vi "Exp1.vi"() -> ()   [LabVIEW 2018]
uses:
  <vilib>/Platform/TimedLoop/XDataNode/timing_clust.ctl
  <vilib>/Platform/TimedLoop/XDataNode/nitl_modes.ctl
  <vilib>/Platform/TimedLoop/XDataNode/wakeup.ctl
  <vilib>/MakerHub/LINX/Public/Peripherals/Analog/Analog Read 1 Chan.vi
  <vilib>/MakerHub/LINX/Public/Peripherals/PWM/PWM Set Duty Cycle 1 Chan.vi
  <vilib>/MakerHub/LINX/Public/Peripherals/Analog/Analog Read N Chans.vi
  <vilib>/MakerHub/LINX/Private/Local IO/LinxAnalogRead.vi
  <vilib>/MakerHub/LINX/Public/Utilities/Check Channel.vi
  <vilib>/MakerHub/LINX/Public/Utilities/Open Serial.vi
  <vilib>/MakerHub/LINX/Private/Utilties/Generate Error.vi
  <vilib>/MakerHub/LINX/Public/Peripherals/PWM/PWM Set Duty Cycle N Chans.vi
  <vilib>/platform/TimedLoop/XDataNode/XDataNode.xnode
  <vilib>/MakerHub/LINX/LMH-LINX.lvlib
  <vilib>/Platform/TimedLoop/XDataNode/XDNodeRunTimeDep.lvlib
panel:
  out "Finished Late? [i-1]":bool
  in  "Duty Cycle (0-100)":dbl min=0.0 max=1.0 step=0.1
  out "Temperature":dbl(graph)=297.8515625
  in  "Stop Button":bool
  in  "Serial Port":refnum<visa-resource-name>="COM4"
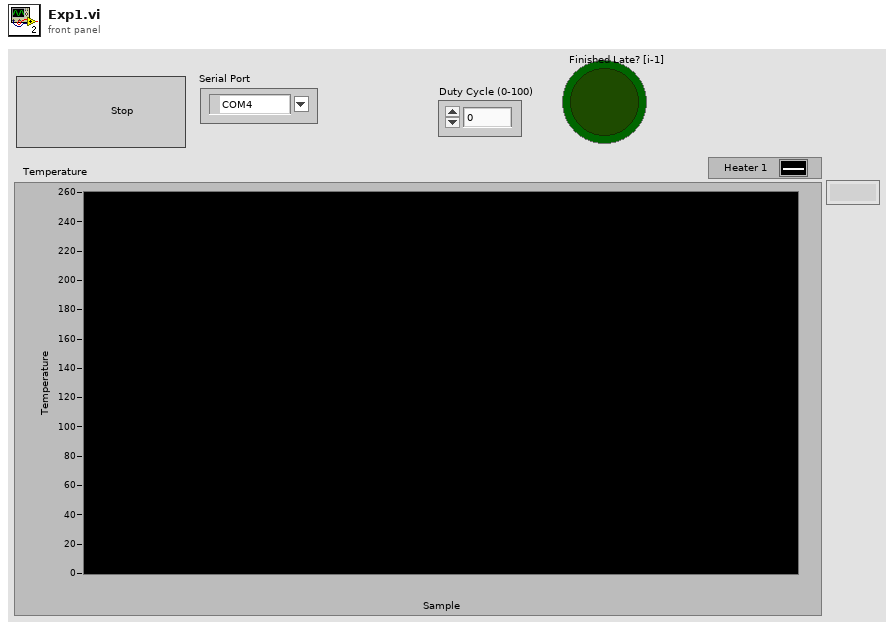
[diagram p1: front panel]
types:
  T1 = enum16{"open", "replace", "create", "open or create", "replace or create", "replace or create with confirmation"}
  T2 = typedef "XDNodeRunTimeDep.lvlib/timing_clust.ctl" = cluster{"Expected End [f-1]":u64, "Actual End [f-1]":u64, "Finished Late? [f-1]":bool, "Expected End [i-1]":u64, "Actual End [i-1]":u64, "Finished Late? [i-1]":bool, "Expected Start [i]":u64, "Actual Start [i]":u64, "Expected Start [f]":u64, "Actual Start [f]":u64, "Source Name":string, "Structure Name":string, "Period":i64, "Deadline":i64, "Offset":i64, "Start":i64, "Priority":i32, "Timeout":i32, "Mode":T3, "Wakeup Reason":T4, "Error":errorcluster, "Source Type":string, "Secondary Source Type":string, "Global End Time":u64, "Global Start Time":u64, "Frame Duration":u64, "Iteration Duration":u64, "Assigned CPU":i32, "I/O Scan Engine Mode":u32}
  T3 = typedef "XDNodeRunTimeDep.lvlib/nitl_modes.ctl" = enum32{"No Change", "Process missed periods, maintain original phase", "Discard missed periods, maintain original phase", "Process missed periods, ignore original phase", "Discard missed periods, ignore original phase"}
  T4 = typedef "XDNodeRunTimeDep.lvlib/wakeup.ctl" = enum32{"Normal", "Aborted", "Asynchronous wakeup", "Timing source error", "Timed loop error", "Timeout"}
  T5 = typedef "LMH-LINX.lvlib/LINX Ref.ctl" = cluster{"IO":T6, "Interface":T7, "LINX Device Config":T8}
  T6 = typedef "LMH-LINX.lvlib/Platform.ctl" = enum16{"Remote", "Local"}
  T7 = typedef "LMH-LINX.lvlib/Interface.ctl" = enum16{"Serial", "TCP"}
  T8 = typedef "LMH-LINX.lvlib/Device.lvlib/LINX Device Config.ctl" = cluster{"Interface":T7, "COM Port":refnum<visa-resource-name>, "TCP Configuration":T9, "Device Family":u8, "Device ID":u8, "Device Name":string, "TCP Ref":refnum<k5>, "Channels":T10}
  T9 = typedef "LMH-LINX.lvlib/Device.lvlib/TCP Config.ctl" = cluster{"IP Address":string, "Port":u16}
  T10 = typedef "LMH-LINX.lvlib/Channels.ctl" = cluster{"DI":u8[], "DO":u8[], "AI":u8[], "AO":u8[], "PWM":u8[], "QE":u8[], "UART":u8[], "I2C 2":u8[], "SPI":u8[], "CAN":u8[], "Servo":u8[], "AI Ref (V)":dbl, "AI Resolution (Bits)":u8, "AO Ref (V)":dbl, "AO Resolution (Bits)":u8}
  T11 = enum16{"big-endian, network order", "native, host order", "little-endian"}
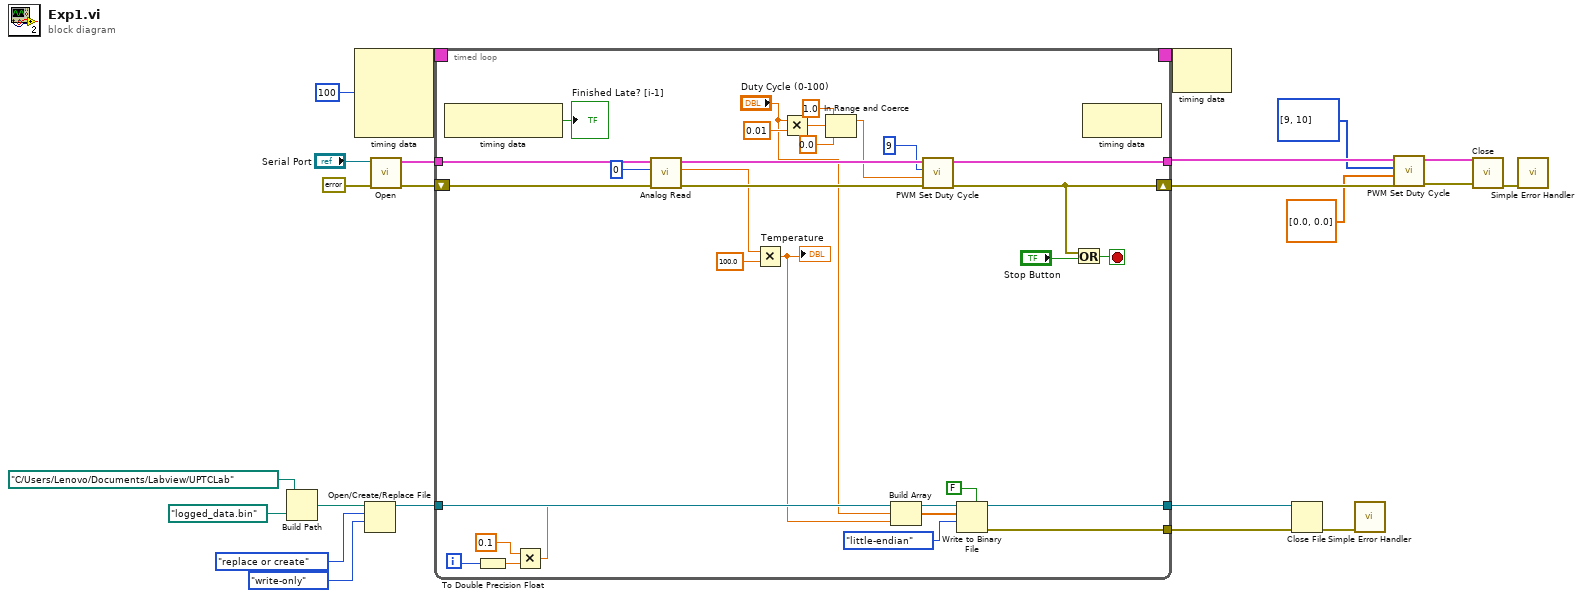
[diagram p0: block diagram]
diagram:
  n1 = Build Path(base path=path "C:/Users/Lenovo/Documents/Labview/UPTCLab", name or relative path=path "logged_data.bin" ("default name")) -> (appended path=w2:path)
  n2 = node-c288(i64 100 ("Period")) -> (w18:T2)  [unwired: 3 in]
  n3 = Open/Create/Replace File(file path (use dialog)=w2, operation (0:open)=T1."replace or create", access (0:read/write)=enum16{"read/write", "read-only", "write-only"}."write-only") -> (refnum out=w6:refnum<file>)  [unwired: 3 in, 2 out]
  n4 = call-poly <vilib>:"Open.vi"("Error In"=errorcluster {"status"=FALSE, "code"=0, "source"=""}, "Serial Port"="Serial Port") -> ("Error Out"=w22:errorcluster, "LINX Resource"=w23:T5)  [unwired: 7 in, 1 out]
  n5 = timed-loop {
    tunnel: w23 -> [w51]
    tunnel: [w46] -> w14
    shift-right: [w45] -> w13
    shift-left: w22 -> [w50]
    timing: w18 -> [_]
    timing-out: [_] -> w17
    tunnel: w6 -> [w36]
    tunnel: [w28] -> w4
    tunnel: [w27] -> w3
    i -> [w35]
    stop <- w53 stop-if-true
    n6 = node-c288() -> (→"Finished Late? [i-1]":bool)  [unwired: 1 in]
    n7 = To Double Precision Float(number=w35) -> (double precision float=w34:dbl)
    n8 = Multiply(x=0.1, y=w34) -> (x*y=w26:dbl)
    n9 = call-poly <vilib>:"Analog Read.vi"("Error In"=w50, "Analog Channel"=u8 0, "LINX Resource"=w51) -> ("Error Out"=w47:errorcluster, "Voltage"=w43:dbl, "LINX Resource"=w48:T5)  [unwired: 5 in, 1 out]
    n10 = Multiply(x=w43, y=100.0) -> (x*y=w32:dbl)
    "Temperature" <- w32
    n11 = Multiply(x="Duty Cycle (0-100)", y=0.01) -> (x*y=w40:dbl)
    n12 = In Range and Coerce(upper limit=1.0, x=w40, lower limit=0.0) -> (coerced(x)=w39:dbl)  [unwired: 1 out]
    n13 = Build Array(w26, "Duty Cycle (0-100)", w32) -> (w31:dbl[])
    n14 = call-poly <vilib>:"PWM Set Duty Cycle.vi"("Error In"=w47, "Duty Cycle (0-1)"=w39, "PWM Channel"=u8 9, "LINX Resource"=w48) -> ("Error Out"=w45:errorcluster, "LINX Resource"=w46:T5)  [unwired: 6 in]
    n15 = Write to Binary File(file (use dialog)=w36, data=w31, 5:FALSE ("prepend array or string size? (T)"), 9:T11."little-endian" ("byte order (0:big-endian, network order)")) -> (refnum out=w28:refnum<file>, error out=w27:errorcluster)  [unwired: 2 in, 1 out]
    n16 = Or(x=w45, y="Stop Button") -> (x .or. y?=w53:bool)
    n17 = node-c288() -> ()  [unwired: 1 in, 1 out]
  }
  n18 = node-c288(w17) -> ()  [unwired: 1 out]
  n19 = Close File(refnum=w4, error in=w3) -> (error out=w5:errorcluster)  [unwired: 1 out]
  n20 = call <vilib>:"Simple Error Handler.vi"("error in (no error)"=w5) -> ()  [unwired: 4 in, 5 out]
  n21 = call-poly <vilib>:"PWM Set Duty Cycle.vi"("Error In"=w13, "Duty Cycles"=dbl[] [0.0, 0.0], "PWM Channels"=u8[] [9, 10], "LINX Resource"=w14) -> ("Error Out"=w12:errorcluster, "LINX Resource"=w15:T5)  [unwired: 6 in]
  n22 = call <vilib>:"Close.vi"("Error In"=w12, "LINX Resource"=w15) -> ("Error Out"=w20:errorcluster)  [unwired: 9 in]
  n23 = call <vilib>:"Simple Error Handler.vi"("error in (no error)"=w20) -> ()  [unwired: 4 in, 5 out]
